vi "Selected HW Detail's.vi"(1 "HW IP":string[](array[string]), 3 "HW Name":string[](array[string]), 7 "HW Name":string, 13 "Write(F)":bool) -> (4 "A HW IP":string, 8 "Selected HW Name":string[](array[string]), 10 "Selected HW IP":string[](array[string]))   [LabVIEW 2021, in "Hardware Selection.lvlib"]
uses:
  Hardware Selection.lvlib
panel:
  out "error out":errorcluster
  in  "error in (no error)":errorcluster
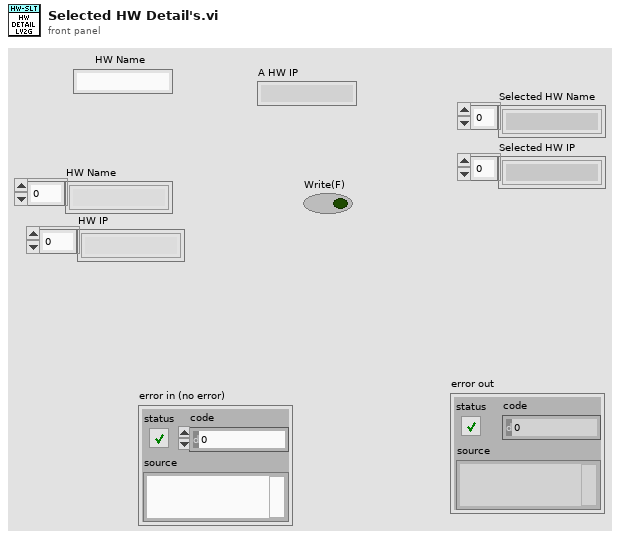
[diagram p1: front panel]
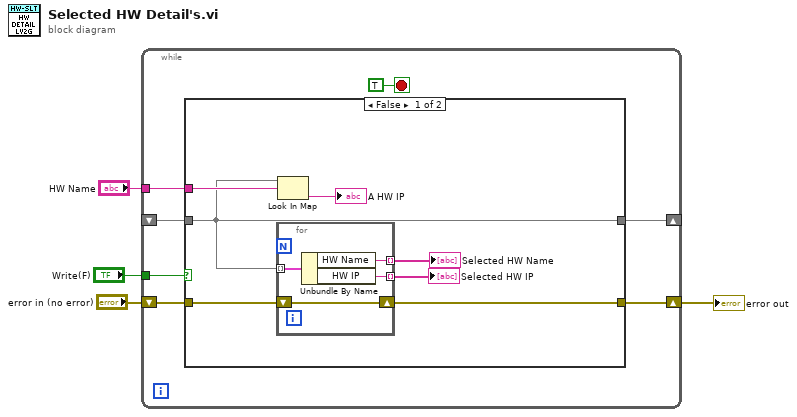
[diagram p0: block diagram]
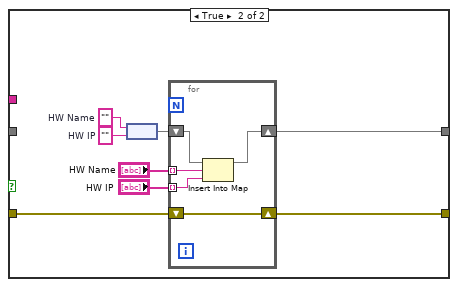
[diagram p2: hidden frame]
diagram:
  n1 = while {
    tunnel: "Write(F)" -> [w11]
    shift-right: [w10] -> w2
    shift-left: "error in (no error)" -> [w9]
    shift-right: [w8] -> _
    shift-left: _ -> [w7]
    tunnel: "HW Name" -> [w6]
    stop <- TRUE stop-if-true
    n2 = case shown="False" w11 {
      tunnel: [w13 w25] -> w10
      tunnel: w9 -> [w12 w24]
      tunnel: [w16 w23] -> w8
      tunnel: w7 -> [w16 _]
      tunnel: w6 -> [w18 _]
      frame False {
        n3 = for {
          tunnel: w16 -> [w22] mode=indexing
          tunnel: [w21] -> w15 mode=indexing
          tunnel: [w20] -> w14 mode=indexing
          shift-right: [w19] -> w13
          shift-left: w12 -> [w19]
          n4 = Unbundle By Name(w22) -> ("HW Name"=w21:string, "HW IP"=w20:string)
        }
        "Selected HW Name" <- w15
        "Selected HW IP" <- w14
        n5 = Look In Map(map=w16, key=w18) -> (value=→"A HW IP":string)  [unwired: 1 in, 1 out]
      }
      frame True {
        w29 = ""  # HW IP
        w30 = ""  # HW Name
        n6 = node(w30, w29) -> (w28:map{string, string})
        n7 = for {
          shift-right: [w34] -> w23
          shift-left: w28 -> [w35]
          tunnel: "HW Name" -> [w33] mode=indexing
          tunnel: "HW IP" -> [w32] mode=indexing
          shift-right: [w31] -> w25
          shift-left: w24 -> [w31]
          n8 = Insert Into Map(map in=w35, key=w33, value=w32) -> (map out=w34:map{string, string})  [unwired: 2 out]
        }
      }
    }
  }
  "error out" <- w2
